vi "Wait for Broadcast.vi"(8 "error in (no error)":errorcluster, 9 "Timeout [ms]":i32, 10 "Broadcast Message":string, 11 "Event Registration Refnum in":refnum<event-registration>) -> (0 "error out":errorcluster, 1 "Stop Received?":bool, 3 "Event Registration Refnum out":refnum<event-registration>)   [LabVIEW 2020, in "Helper Loop.lvclass"]
uses:
  Helper Loop.lvclass
  Process/Protected/Broadcasting/Broadcast Message Cluster.ctl
  Broadcast Event Helpers/Broadcast Event Helpers.lvlib
  Process/Process.lvclass
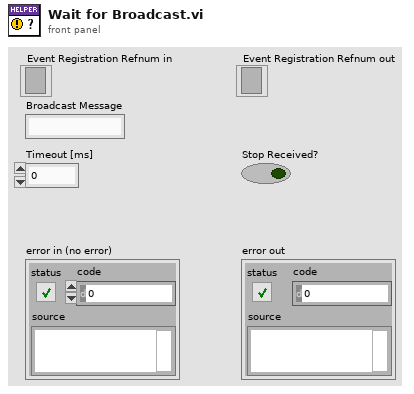
[diagram p1: front panel]
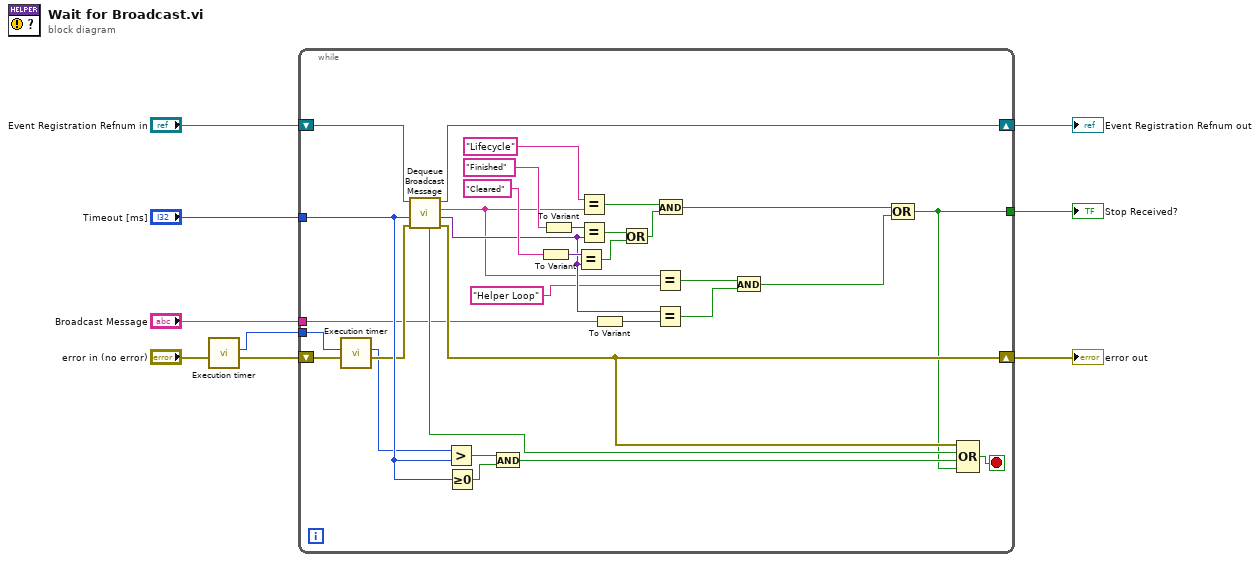
[diagram p0: block diagram]
diagram:
  n1 = call "Execution timer.vi"("error in (no error)"="error in (no error)") -> ("error out"=w2:errorcluster, "Current or Duration [ms]"=w3:u32)  [unwired: 9 in]
  n2 = while {
    tunnel: [w24] -> w9
    tunnel: "Timeout [ms]" -> [w35]
    shift-right: [w40] -> w5
    shift-left: "Event Registration Refnum in" -> [w41]
    shift-right: [w31] -> w4
    shift-left: w2 -> [w39]
    tunnel: w3 -> [w33]
    tunnel: "Broadcast Message" -> [w10]
    stop <- w38 stop-if-true
    n3 = call "Execution timer.vi"("error in (no error)"=w39, "millisecond timer value"=w33) -> ("error out"=w34:errorcluster, "Current or Duration [ms]"=w32:u32)  [unwired: 8 in]
    n4 = call "Dequeue Broadcast Message.vi"("error in (no error)"=w34, "Timeout (-1)"=w35, "Event Registration Refnum"=w41) -> ("error out"=w31:errorcluster, "Message Data"=w17:variant, "Message"=w13:string, "Event Registration Refnum Out"=w40:refnum<event-registration>, "Timed Out?"=w26:bool)  [unwired: 3 in, 1 out]
    n5 = Greater?(x=w32, y=w35) -> (0:w37:bool)
    n6 = Greater Or Equal To 0?(x=w35) -> (x >= 0?=w36:bool)
    n7 = And(x=w37, y=w36) -> (x .and. y?=w25:bool)
    n8 = To Variant(anything="Cleared" ("Message")) -> (Variant=w22:variant)
    n9 = To Variant(anything="Finished" ("Message")) -> (Variant=w27:variant)
    n10 = Equal?(x=w22, y=w17) -> (x = y?=w20:bool)
    n11 = Equal?(x="Lifecycle" ("Message"), y=w13) -> (x = y?=w30:bool)
    n12 = Equal?(x=w27, y=w17) -> (x = y?=w29:bool)
    n13 = To Variant(anything=w10) -> (Variant=w16:variant)
    n14 = Or(x=w29, y=w20) -> (x .or. y?=w21:bool)
    n15 = Equal?(x=w13, y="Helper Loop" ("Message")) -> (x = y?=w11:bool)
    n16 = Equal?(x=w17, y=w16) -> (x = y?=w15:bool)
    n17 = And(x=w30, y=w21) -> (x .and. y?=w23:bool)
    n18 = And(x=w11, y=w15) -> (x .and. y?=w14:bool)
    n19 = Compound Arithmetic op=OR(w23, w14) -> (w24:bool)
    n20 = Compound Arithmetic op=OR(w31, w26, w25, w24) -> (w38:bool)
  }
  "Stop Received?" <- w9
  "error out" <- w4
  "Event Registration Refnum out" <- w5
